vi "Keithley 2001 Select Active Terminals.vi"(8 "error in":T1, 10 "Enum":enum16{"Front", "Rear"}(ring), 11 "GPIB address":string="16") -> (0 "error out":T1, 3 "GPIB address out":string="16")   [LabVIEW 2016]
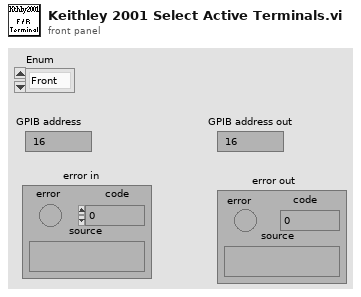
[diagram p1: front panel]
types:
  T1 = cluster{"error":bool, "code":i32, "source":string}
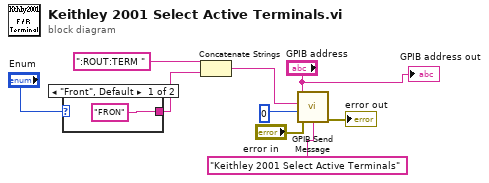
[diagram p0: block diagram]
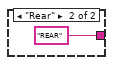
[diagram p2: hidden frame]
diagram:
  n1 = case shown="\"Front\", Default" "Enum" {
    tunnel: ["FRON" "REAR"] -> w3
    frame "Front", Default {
    }
    frame "Rear" {
    }
  }
  n2 = Concatenate Strings(":ROUT:TERM ", w3) -> (w2:string)
  n3 = call <instrlib>:"GPIB Send Message.vi"("address string"="GPIB address", "write buffer"=w2, "source"="Keithley 2001 Select Active Terminals", "write mode (set END:0)"=0, "error in"="error in") -> ("error out"=→"error out":T1)  [unwired: 2 in, 2 out]
  "GPIB address out" <- "GPIB address"
